vi "XY Graph Add Data to Last Plots.vi"(8 "error in (no error)":errorcluster, 9 "First Abscissa (0)":i32, 10 "Plots Data Array":dbl[][](array[numeric]), 11 "XYGraph in":refnum<vi>) -> (0 "error out":errorcluster)   [LabVIEW 2021, in "XY Graph Add-Ons.lvlib"]
doc: "Adds data points to the last plots in a graph.\n\nProvide a N x M array of data, where N in the number of elements in the series and M is the number of plots."
uses:
  XY Graph Add-Ons.lvlib
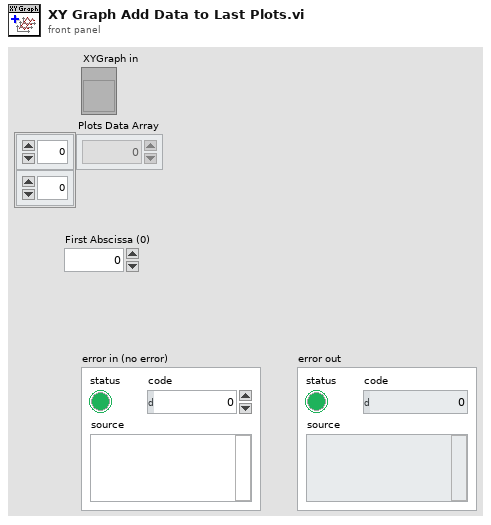
[diagram p1: front panel]
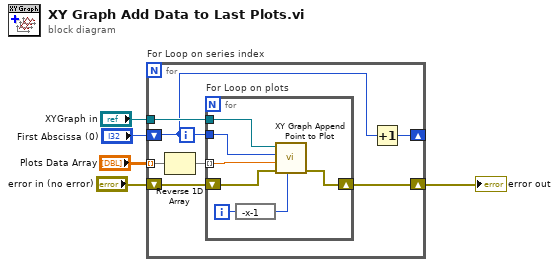
[diagram p0: block diagram]
diagram:
  n1 = for "For Loop on series index" {
    tunnel: "XYGraph in" -> [w10]
    tunnel: "Plots Data Array" -> [w9] mode=indexing
    shift-right: [w12] -> w5
    shift-left: "error in (no error)" -> [w11]
    shift-right: [w6] -> _
    shift-left: "First Abscissa (0)" -> [w7]
    n2 = Reverse 1D Array(array=w9) -> (reversed array=w8:dbl[])
    n3 = for "For Loop on plots" {
      tunnel: w8 -> [w19] mode=indexing
      tunnel: w10 -> [w17]
      tunnel: w7 -> [w15]
      shift-right: [w13] -> w12
      shift-left: w11 -> [w14]
      i -> [w16]
      n4 = expression code="-x-1"(w16) -> (w18:i32)
      n5 = call "XY Graph Append Point to Plot.vi"("Plot ID (-1: last)"=w18, "error in (no error)"=w14, "y"=w19, "x"=w15, "XYGraph in"=w17) -> ("error out"=w13:errorcluster)  [unwired: 3 in, 3 out]
    }
    n6 = Increment(x=w7) -> (x+1=w6:i32)
  }
  "error out" <- w5
